vi "Get Shoot Cube Command.vi"(8 "Height Preset":T2=enum."High", 9 "Deadband":dbl=0.2 format="%#_13g", 10 "Driver Buttons":bool[](array[boolean]), 11 "Driver Axes":dbl[](array[numeric])) -> (3 "Shoot Cube Preset":cluster{"Shot Preset":T1})   [LabVIEW 2020]
uses:
  manipulator/Implementation/Typedefs/Cascade Height.ctl
  manipulator/Implementation/Typedefs/Cube Shooting Presets.ctl
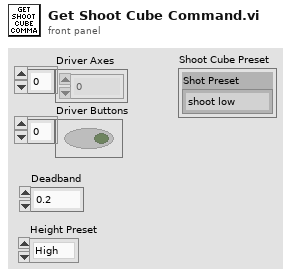
[diagram p1: front panel]
types:
  T1 = typedef "Cube Shooting Presets.ctl" = enum16{"shoot low", "shoot mid", "shoot high"}
  T2 = typedef "Cascade Height.ctl" = enum16{"Middle", "High"}
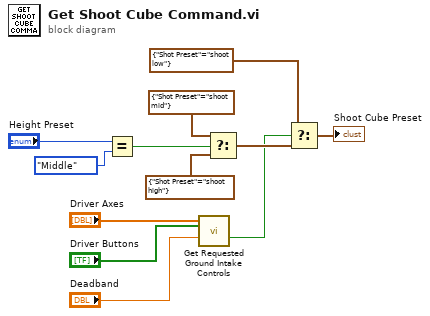
[diagram p0: block diagram]
diagram:
  n1 = Equal?(x="Height Preset", y=Cascade_Height."Middle") -> (x = y?=w12:bool)
  n2 = call "Get Requested Ground Intake Controls.vi"("Driver Axes"="Driver Axes", "Driver Buttons"="Driver Buttons", "Deadband"="Deadband") -> ("Outtake Requested?"=w6:bool)  [unwired: 6 in, 6 out]
  n3 = Select(t=cluster{"Shot Preset":T1} {"Shot Preset"=enum."shoot mid"} ("Shoot Cube Parameters"), s=w12, f=cluster{"Shot Preset":T1} {"Shot Preset"=enum."shoot high"} ("Shoot Cube Parameters")) -> (s? t:f=w7:cluster{"Shot Preset":T1})
  n4 = Select(t=cluster{"Shot Preset":T1} {"Shot Preset"=enum."shoot low"}, s=w6, f=w7) -> (s? t:f=→"Shoot Cube Preset":cluster{"Shot Preset":T1})
